vi "LOGIC_gbls.vi"() -> ()   [LabVIEW 2016]
uses:
  DBSHAND/private/vis/DatabaseHand_RefNum.ctl
panel:
  out "LOGIC_DatabaseRef":T1
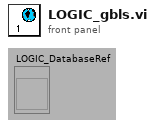
[diagram p1: front panel]
types:
  T1 = typedef "DatabaseHand_RefNum.ctl" = refnum<vi>
diagram:
